vi "path globals.vi"() -> ()   [LabVIEW 2013, in "Linux RT IPC.C.lvlib"]
uses:
  Linux RT IPC.C.lvlib
panel:
  in  "librt path":path=path "/lib/librt.so.1"
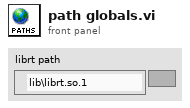
[diagram p1: front panel]
diagram:
